vi "Simple Reader.vi"(8 "error in (no error)":errorcluster, 11 "Quantum Design Driver in":refnum<class "Quantum Design Driver.lvclass">) -> (0 "error out":errorcluster, 2 "Signals":dbl[](array[numeric]), 3 "Quantum Design Driver out":refnum<class "Quantum Design Driver.lvclass">)   [LabVIEW 2018, in "Quantum Design Driver.lvclass"]
uses:
  Quantum Design Driver.lvclass
  Quantum Design Driver.lvclass/Quantum Design Driver.ctl
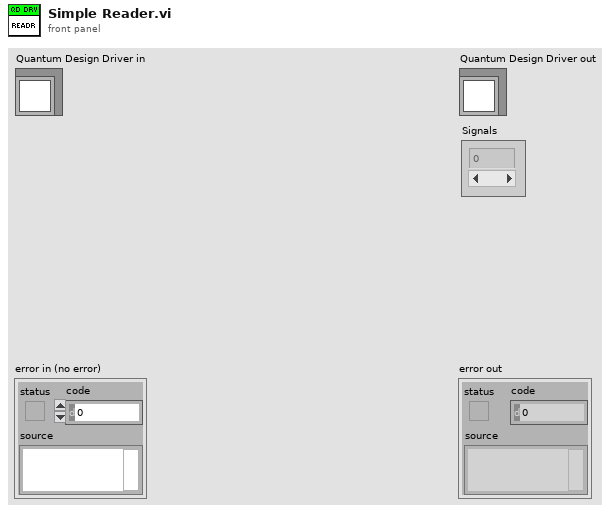
[diagram p1: front panel]
types:
  T1 = typedef "Quantum Desing Configuration.ctl" = cluster{"Address":string, "Instrument type":u16, "Remote":bool, "Measurements":enum16{"Temperature", "Field", "Position"}[]}
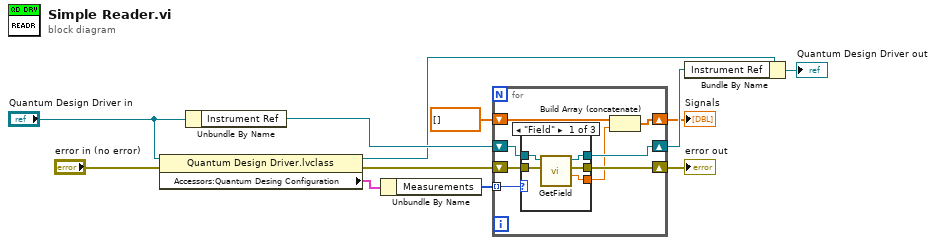
[diagram p0: block diagram]
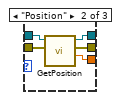
[diagram p2: hidden frame]
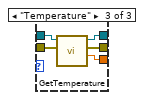
[diagram p3: hidden frame]
diagram:
  n1 = property class="Quantum Design Driver.lvclass"(reference="Quantum Design Driver in", error in="error in (no error)") -> (reference out=w8:refnum<class "Quantum Design Driver.lvclass">, error out=w5:errorcluster, "Accessors:Quantum Desing Configuration"=w11:T1)
  n2 = Unbundle By Name("Quantum Design Driver in") -> ("Instrument Ref"=w10:refnum<k24>)
  n3 = Unbundle By Name(w11) -> ("Measurements"=w6:enum16{"Temperature", "Field", "Position"}[])
  n4 = for {
    tunnel: w6 -> [w16] mode=indexing
    shift-right: [w13] -> w1
    shift-left: dbl[] [] -> [w15]
    shift-right: [w17] -> w3
    shift-left: w5 -> [w20]
    shift-right: [w18] -> w4
    shift-left: w10 -> [w19]
    n5 = case shown="\"Field\"" w16 {
      tunnel: w20 -> [w25 w30 w35]
      tunnel: w19 -> [w24 w29 w34]
      tunnel: [w23 w28 w33] -> w18
      tunnel: [w22 w27 w32] -> w17
      tunnel: [w21 w26 w31] -> w14
      frame "Field" {
        n6 = call <instrlib>:"GetField.vi"("error in (no error)"=w25, "Instrument Ref In"=w24) -> ("Field"=w21:dbl, "error out"=w22:errorcluster, "Instrument Ref Out"=w23:refnum<k24>)  [unwired: 3 in, 2 out]
      }
      frame "Position" {
        n7 = call <instrlib>:"GetPosition.vi"("error in (no error)"=w30, "Instrument Ref In"=w29) -> ("Position"=w26:dbl, "error out"=w27:errorcluster, "Instrument Ref Out"=w28:refnum<k24>)  [unwired: 2 in, 1 out]
      }
      frame "Temperature" {
        n8 = call <instrlib>:"GetTemperature.vi"("error in (no error)"=w35, "Instrument Ref In"=w34) -> ("Temperature"=w31:dbl, "error out"=w32:errorcluster, "Instrument Ref Out"=w33:refnum<k24>)  [unwired: 3 in, 2 out]
      }
    }
    n9 = Build Array (concatenate)(w15, w14) -> (w13:dbl[])
  }
  "error out" <- w3
  "Signals" <- w1
  n10 = Bundle By Name(cluster=w8, "Instrument Ref"=w4) -> (→"Quantum Design Driver out":refnum<class "Quantum Design Driver.lvclass">)
